vi "I2C Utility Example EEPROM Write.vi"() -> ()   [LabVIEW 2020]
panel:
  out "I2C COM Error Out":errorcluster={"status"=FALSE, "code"=0, "source"="No Error"}
  in  "I2C_NUM_BYTES_RX":i32
  in  "I2C_WRITE_DATA":u8[](array[numeric])=[0, 222, 173, 190, 239, 1, 2, 3, 4, 5, 6, 7, 222, 173, 190, 239] format="%x"
  out "I2C_READ_DATA":u8[](array[numeric]) format="%x"
  out "Acks Received":dbl
  in  "I2C_SLAVE_ADDRESS":i32=80
  in  "I2C_OPTIONS":i32
  in  "I2C_SPEED_THROTTLE":i32
  in  "I2C_SCL_DIONUM":i32=1
  in  "I2C_SDA_DIONUM":i32
  out "Error String":string="No Error"
  out "error out":errorcluster
  out "ConnectionType Out":i32
  out "DeviceType Out":i32
  in  "Identifier":string="LJM_idANY"
  in  "ConnectionType":string="LJM_ctANY"
  in  "DeviceType":string="LJM_dtANY"
  # "Before running this program:\n1. Attach a LJTick-DAC to FIO0 and FIO1\n2. Configure Device Opening Settings (DeviceType, ConnectionType, and Identifier)\n3. Configure I2C Settings (I2C_SDA_DIONUM, I2C_SCL_DIONUM, I2C_SPEED_THROTTLE, I2C_OPTIONS, I2C_SLAVE_ADDRESS)\n4. Run the .vi by either 'ctrl+r' or by pressing the \"Run\" button.\n\nThis program interfaces with the Microchip 24C01C EEPROM built into the LJTick-DAC, it has a Slave Address of 0x50 or d80.  \nThis program lets you write and read data to/from the EEPROM.  It uses the \"I2C Utility.vi\" to configure and control a LabJack T7's \nI2C functionality.   It is important to note that this EEPROM lets you perform page read's and writes of 1-15 bytes of data.  This\nprogram does not check that limitation and report an error, you have been warned!\n\nBy default the program configures the LabJack to write  0-15 bytes of data to the EEPROM starting at page (PageNum).  \nWhen the .vi is run the LabJack:\n1. Sends a Start I2C command\n2. Sends the Slave Address followed by a write bit (0)\n3. Waits for an Ack from the EEPROM\n4. Writes the remaining bytes of data while waiting for Acks.\n\nThings that can be configured:\n1. You can configure the starting Page to write to by changing the PageNum value in the \"I2C_WRITE_DATA\" array.\n2. You can configure how many values to write by declaring/deleting elements from the \"I2C_WRITE_DATA\" array.\n    Right click on array, \"Data Operations\"->\"Delete Element\" or \"Insert Element Before\".\n3. You can configure how many bytes are read after data is written.  Is 0  default in this mode so that data is only written."
  # "Device Opening Settings"
  # "PageNum"
  # "Data [0]"
  # "Data [0]"
  # "Data [1]"
  # "Data [2]"
  # "Data [1]"
  # "Data [2]"
  # "Data [3]"
  # "Data [3]"
  # "..."
  # "..."
  # "I2C Settings"
  # "Configures the FIO channel that the \nSDA signal should appear on."
  # "Configures the FIO channel that the \nSDA signal should appear on."
  # "Configures the I2C Clock Speed\n (frequency)"
  # "Configures the I2C options"
  # "..."
  # "Data [14]"
  # "..."
  # "Configure the slave address to be sent \nat the start of each data transfer"
  # "Data [14]"
  # "Errors:"
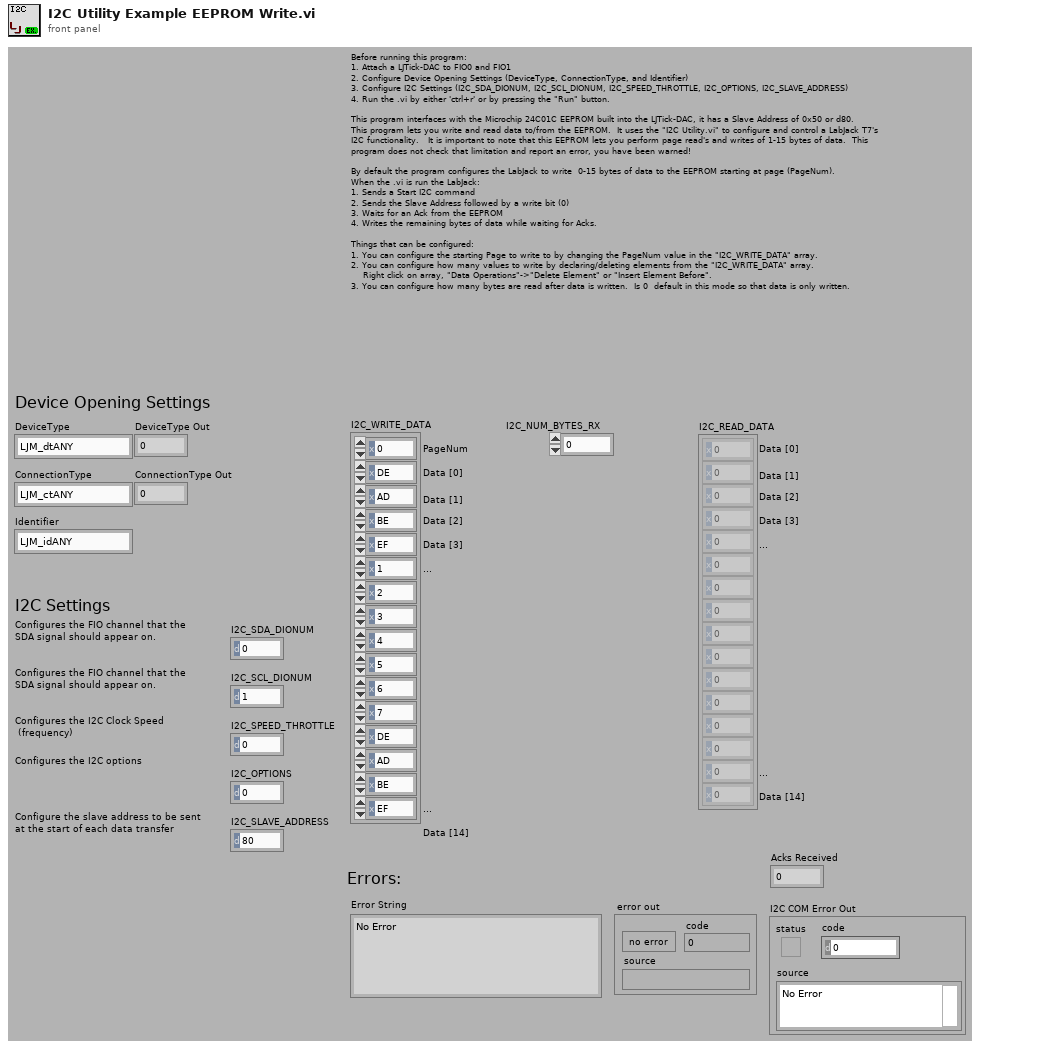
[diagram p1: front panel]
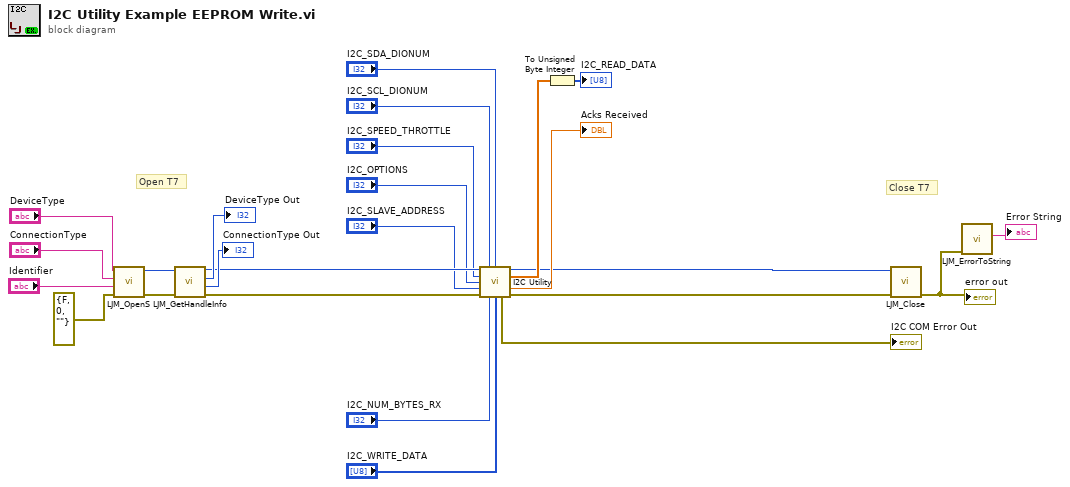
[diagram p0: block diagram]
diagram:
  # "Close T7"
  # "Open T7"
  n1 = call "LJM_OpenS.vi"("error in"=errorcluster {"status"=FALSE, "code"=0, "source"=""} ("error in (no error)"), "Identifier"="Identifier", "ConnectionType"="ConnectionType", "DeviceType"="DeviceType") -> ("error out"=w24:errorcluster, "Handle"=w23:i32)  [unwired: 6 in]
  n2 = call "LJM_GetHandleInfo.vi"("error in"=w24, "Handle In"=w23) -> ("error out"=w14:errorcluster, "ConnectionType"=→"ConnectionType Out":i32, "DeviceType"=→"DeviceType Out":i32, "Handle Out"=w15:i32)  [unwired: 2 in, 4 out]
  n3 = call "I2C Utility.vi"("Handle In"=w15, "I2C_SDA_DIONUM"="I2C_SCL_DIONUM", "I2C_SCL_DIONUM"="I2C_SDA_DIONUM", "I2C_SPEED_THROTTLE"="I2C_SPEED_THROTTLE", "I2C_OPTIONS"="I2C_OPTIONS", "I2C_SLAVE_ADDRESS"="I2C_SLAVE_ADDRESS", "error in"=w14, "I2C_NUM_BYTES_RX"="I2C_NUM_BYTES_RX", "I2C_WRITE_DATA"="I2C_WRITE_DATA") -> ("Handle Out"=w6:i32, "Data Read"=w8:dbl[], "Acks Received"=→"Acks Received":dbl, "I2C COM Error Out"=→"I2C COM Error Out":errorcluster, "error out"=w5:errorcluster)  [unwired: 2 in]
  n4 = To Unsigned Byte Integer(number=w8) -> (unsigned 8bit integer=→"I2C_READ_DATA":u8[])
  n5 = call "LJM_Close.vi"("error in"=w5, "Handle"=w6) -> ("error out"=w17:errorcluster)  [unwired: 9 in]
  "error out" <- w17
  n6 = call "LJM_ErrorToString.vi"("error in"=w17) -> ("String"=→"Error String":string)  [unwired: 10 in]
